vi "store variable.vi"(8 "error in":errorcluster, 9 "varient in":variant, 11 "refnum in":T1) -> (0 "error out":errorcluster, 2 "Variable Name":string, 3 "refnum out":T1)   [LabVIEW 2020, in "Publisher Subscriber.lvlib"]
uses:
  Publisher Subscriber.lvlib
  Controls/node refnum.ctl
  Controls/node dvr data.ctl
  Controls/data cluster.ctl
  Controls/subscription bank ref.ctl
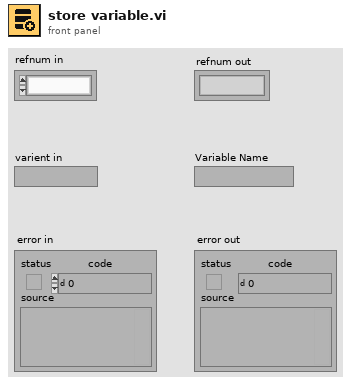
[diagram p1: front panel]
types:
  T1 = typedef "Publisher Subscriber.lvlib/node refnum.ctl" = refnum<k1>
  T2 = typedef "Publisher Subscriber.lvlib/node dvr data.ctl" = cluster{"queue ref":refnum<queue>, "Subscription Bank Ref":refnum<data-value>, "Command":string, "Data":variant, "Subscriptions []":set{string}, "Variables DVR Ref":refnum<data-value>}
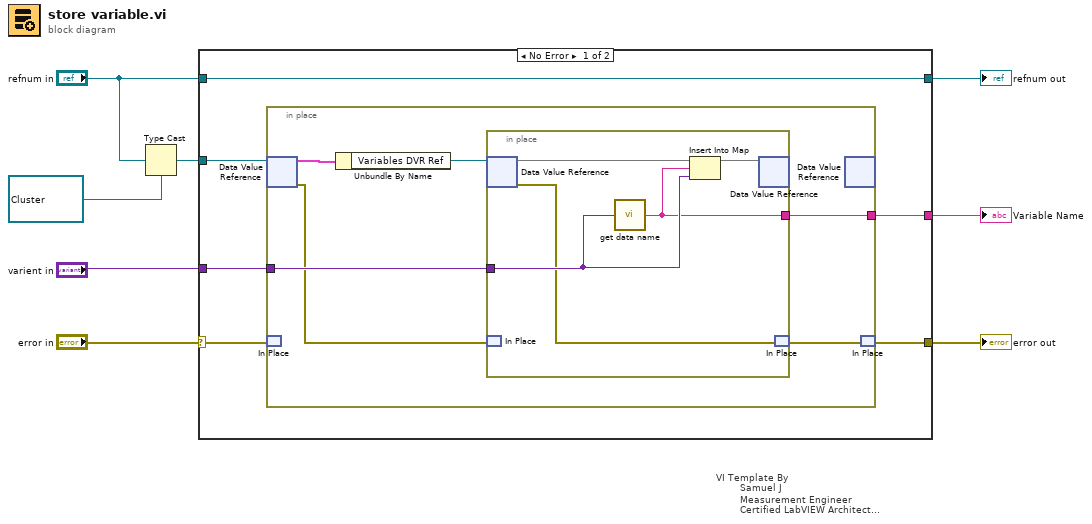
[diagram p0: block diagram]
diagram:
  n1 = Type Cast(type=refnum<data-value> refnum ("data value reference"), x="refnum in") -> (*(type *) &x=w5:refnum<data-value>)
  n2 = case "VI Template By\n        Samuel J\n        Measurement Engineer\n        Certified LabVIEW Architect\n        Vestas Technology R&D Chennai" shown="No Error" "error in" {
    selector: "error in" -> [w12 w27]
    tunnel: [w11 w27] -> w7
    tunnel: w5 -> [w13 _]
    tunnel: [w14 w26] -> w4
    tunnel: "refnum in" -> [w14 w26]
    tunnel: "varient in" -> [w10 _]
    tunnel: [w9 _] -> w1
    frame No Error {
      n3 = in-place {
        in-place-border: w10 -> [w18]
        in-place-border: [w15] -> w9
        n4 = in-place-dvr #1(w13) -> (w20:T2, w17:errorcluster)
        n5 = in-place-match #2(w12) -> ()  [unwired: 1 out]
        n6 = Unbundle By Name(w20) -> ("Variables DVR Ref"=w19:refnum<data-value>)
        n7 = in-place {
          in-place-border: w18 -> [w23]
          in-place-border: [w21] -> w15
          n8 = in-place-dvr #3(w19) -> (w25:map{string, variant}, w22:errorcluster)
          n9 = in-place-match #4(w17) -> ()  [unwired: 1 out]
          n10 = call "get data name.vi"("data in"=w23) -> ("Name"=w21:string)
          n11 = Insert Into Map(map in=w25, key=w21, value=w23) -> (map out=w24:map{string, variant})  [unwired: 2 out]
          n12 = in-place-dvr #3(w24) -> ()  [unwired: 2 out]
          n13 = in-place-match #4(w22) -> (w16:errorcluster)
        }
        n14 = in-place-dvr #1() -> ()  [unwired: 1 in, 2 out]
        n15 = in-place-match #2(w16) -> (w11:errorcluster)
      }
    }
    frame Error {
    }
  }
  "error out" <- w7
  "refnum out" <- w4
  "Variable Name" <- w1
